vi "Send error.vi"(8 "error in (no error)":errorcluster, 10 "Error":errorcluster, 11 "IUnregister in":refnum<class "IUnregister.lvclass">) -> (0 "error out":errorcluster, 3 "IUnregister out":refnum<class "IUnregister.lvclass">)   [LabVIEW 2020, in "wamplv.lvlib" / "IUnregister.lvclass"]
uses:
  IUnregister.lvclass
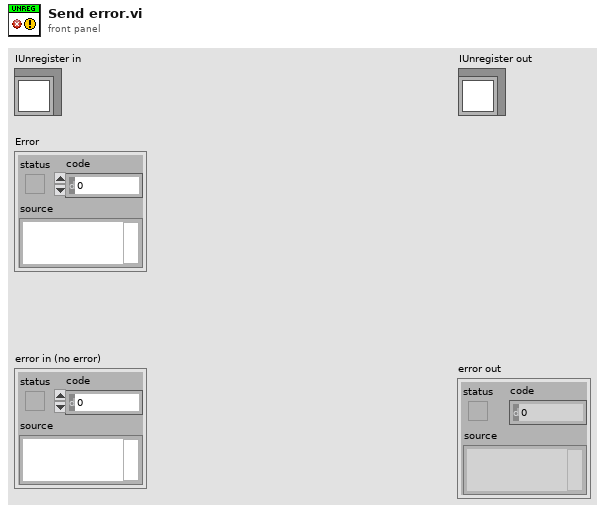
[diagram p1: front panel]
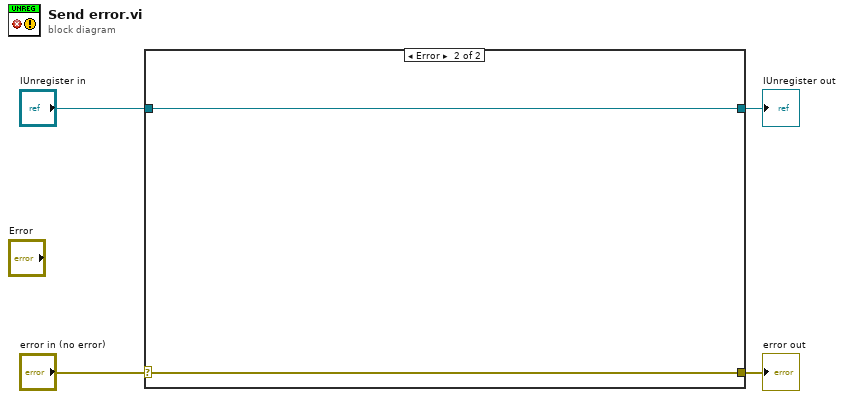
[diagram p0: block diagram]
diagram:
  n1 = case shown="Error" "error in (no error)" {
    selector: "error in (no error)" -> [w5 w8]
    tunnel: [w5 w8] -> w3
    tunnel: [w6 w7] -> w1
    tunnel: "IUnregister in" -> [w6 w7]
    frame No Error {
      # "Wire the error cluster across even in the \"No Error\"\ncase so that warnings get propagated."
    }
    frame Error {
    }
  }
  "error out" <- w3
  "IUnregister out" <- w1
